vi "methane_reactor_setup.vi"() -> (2 "spec_file":path)   [LabVIEW 2019]
uses:
  lib/libSimulationControl/libSimulationControl.lvlib
  lib/libCheckpointUpdate/libCheckpointUpdate.lvlib
panel:
  # "*******************************************************************\nBiogas Plant Control\n\nAuthor: Paul Zügel\nGCSC-Frankfurt am Main 2020\n\n*******************************************************************"
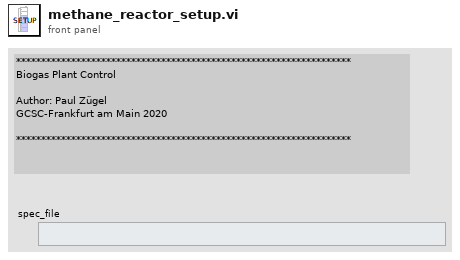
[diagram p1: front panel]
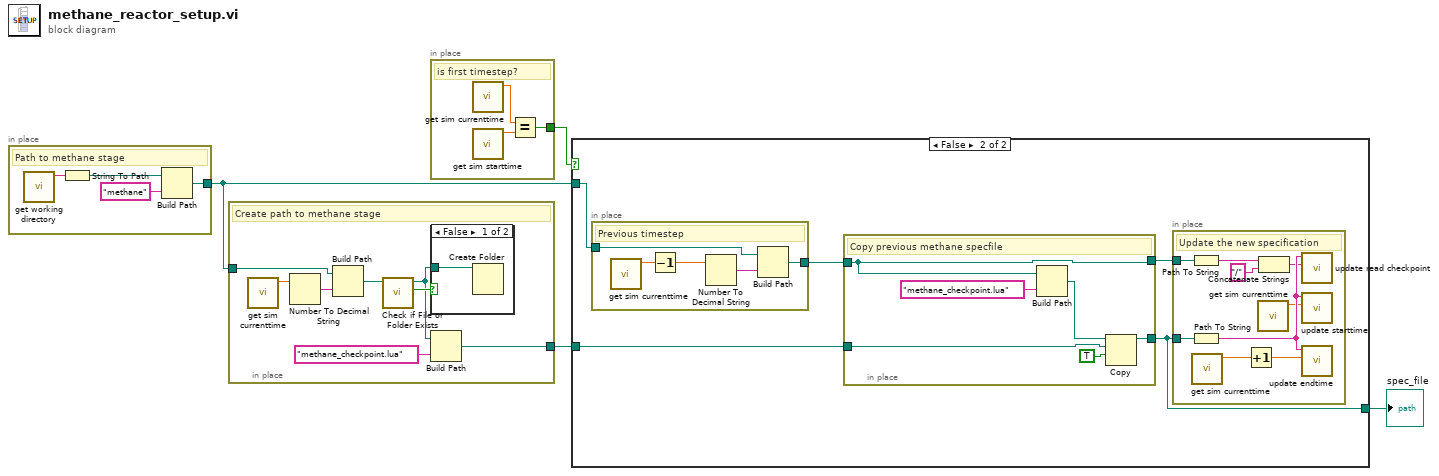
[diagram p0: block diagram]
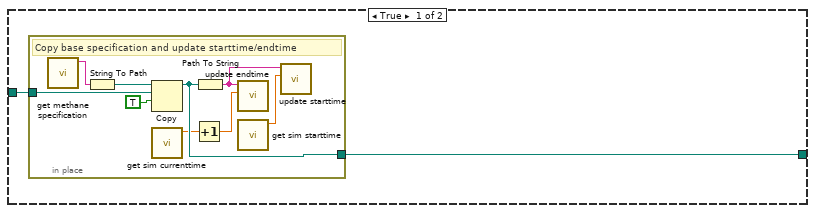
[diagram p3: hidden frame]
diagram:
  n1 = in-place {
    in-place-border: [w7] -> w2
    # "Path to methane stage"
    n2 = call "get working directory.vi"() -> ("function return"=w8:string)  [unwired: 10 in, 1 out]
    n3 = String To Path(string=w8) -> (path=w5:path)
    n4 = Build Path(base path=w5, name or relative path="methane" ("string")) -> (appended path=w7:path)
  }
  n5 = in-place {
    in-place-border: [w11] -> w1
    in-place-border: w2 -> [w9]
    # "Create path to methane stage"
    n6 = call "get sim currenttime.vi"() -> ("current_time"=w10:dbl)  [unwired: 10 in, 1 out]
    n7 = Number To Decimal String(number=w10) -> (decimal integer string=w15:string)  [unwired: 1 in]
    n8 = Build Path(base path=w9, name or relative path=w15) -> (appended path=w14:path)
    n9 = call <vilib>:"Check if File or Folder Exists.vi"("path"=w14) -> ("file or folder exists?"=w16:bool, "dup path"=w13:path)  [unwired: 8 in, 1 out]
    n10 = case shown="False" w16 {
      tunnel: w13 -> [w17 _]
      frame False {
        n11 = Create Folder(path (use dialog)=w17) -> ()  [unwired: 2 in, 3 out]
      }
      frame True {
      }
    }
    n12 = Build Path(base path=w13, name or relative path="methane_checkpoint.lua" ("string")) -> (appended path=w11:path)
  }
  n13 = in-place {
    in-place-border: [w20] -> w4
    # "is first timestep?"
    n14 = call "get sim currenttime.vi"() -> ("current_time"=w18:dbl)  [unwired: 10 in, 1 out]
    n15 = call "get sim starttime.vi"() -> ("sim_starttime"=w19:dbl)  [unwired: 10 in, 1 out]
    n16 = Equal?(x=w18, y=w19) -> (x = y?=w20:bool)
  }
  n17 = case shown="False" w4 {
    tunnel: w2 -> [_ w36]
    tunnel: [w22 w32] -> w3
    tunnel: w1 -> [w21 w33]
    frame True {
      n18 = in-place {
        in-place-border: [w29] -> w22
        in-place-border: w21 -> [w28]
        # "Copy base specification and update starttime/endtime"
        n19 = call "get methane specification.vi"() -> ("function return"=w31:string)  [unwired: 10 in, 1 out]
        n20 = String To Path(string=w31) -> (path=w30:path)
        n21 = Copy(9:TRUE ("overwrite (F)"), 10:w28, 11:w30) -> (3:w29:path)  [unwired: 2 in, 2 out]
        n22 = call "get sim currenttime.vi"() -> ("current_time"=w24:dbl)  [unwired: 10 in, 1 out]
        n23 = Increment(x=w24) -> (x+1=w23:dbl)
        n24 = Path To String(path=w29) -> (string=w25:string)
        n25 = call "update endtime.vi"("endtime"=w23, "spec_dir"=w25) -> ()  [unwired: 9 in, 1 out]
        n26 = call "get sim starttime.vi"() -> ("sim_starttime"=w26:dbl)  [unwired: 10 in, 1 out]
        n27 = call "update starttime.vi"("starttime"=w26, "spec_dir"=w25) -> ()  [unwired: 9 in, 1 out]
      }
    }
    frame False {
      n28 = in-place {
        in-place-border: w36 -> [w55]
        in-place-border: [w53] -> w35
        # "Previous timestep"
        n29 = call "get sim currenttime.vi"() -> ("current_time"=w52:dbl)  [unwired: 10 in, 1 out]
        n30 = Decrement(x=w52) -> (x-1=w56:dbl)
        n31 = Number To Decimal String(number=w56) -> (decimal integer string=w54:string)  [unwired: 1 in]
        n32 = Build Path(base path=w55, name or relative path=w54) -> (appended path=w53:path)
      }
      n33 = in-place {
        in-place-border: w35 -> [w38]
        in-place-border: w33 -> [w41]
        in-place-border: [w38] -> w34
        in-place-border: [w37] -> w32
        # "Copy previous methane specfile"
        n34 = Build Path(base path=w38, name or relative path="methane_checkpoint.lua" ("string")) -> (appended path=w40:path)
        n35 = Copy(9:TRUE ("overwrite (F)"), 10:w41, 11:w40) -> (3:w37:path)  [unwired: 2 in, 2 out]
      }
      n36 = in-place {
        in-place-border: w32 -> [w51]
        in-place-border: w34 -> [w46]
        # "Update the new specification"
        n37 = Path To String(path=w46) -> (string=w49:string)
        n38 = Path To String(path=w51) -> (string=w50:string)
        n39 = call "get sim currenttime.vi"() -> ("current_time"=w44:dbl)  [unwired: 10 in, 1 out]
        n40 = Increment(x=w44) -> (x+1=w43:dbl)
        n41 = call "get sim currenttime.vi"() -> ("current_time"=w45:dbl)  [unwired: 10 in, 1 out]
        n42 = Concatenate Strings(w49, "/" ("string")) -> (w47:string)
        n43 = call "update read checkpoint.vi"("checkpoint_dir"=w47, "spec_dir"=w50) -> ()  [unwired: 9 in, 1 out]
        n44 = call "update starttime.vi"("starttime"=w45, "spec_dir"=w50) -> ()  [unwired: 9 in, 1 out]
        n45 = call "update endtime.vi"("endtime"=w43, "spec_dir"=w50) -> ()  [unwired: 9 in, 1 out]
      }
    }
  }
  "spec_file" <- w3
